vi "test_CCDSetAndGetTriggerIn.vi"(7 "Test should pass":bool=TRUE, 8 "error in":errorcluster, 9 "tear down connection":bool=TRUE, 10 "set-up a connection":bool=TRUE, 11 "device selection":enum16{"monochromator", "CCD", "SCD"}(ring)=enum."CCD") -> (0 "error out":errorcluster)   [LabVIEW 2023]
uses:
  <vilib>/addons/_JKI Toolkits/Caraya/classes/Test/Test.lvclass
  <vilib>/addons/_JKI Toolkits/Caraya/classes/Assert/Assert.lvclass
  <vilib>/addons/_JKI Toolkits/Caraya/classes/Assert/Assert Not Error.vi
  <vilib>/addons/_JKI Toolkits/Caraya/classes/Assert/Assert Equal Value and Type_Variant.vi
  Classes/CCD/CCD.lvclass
  Classes/CCD/TriggerInAddressRing.ctl
  Classes/CCD/TriggerInEventRing.ctl
  Classes/CCD/TriggerInSignalTypeRing.ctl
panel:
  # "Connector Pane"
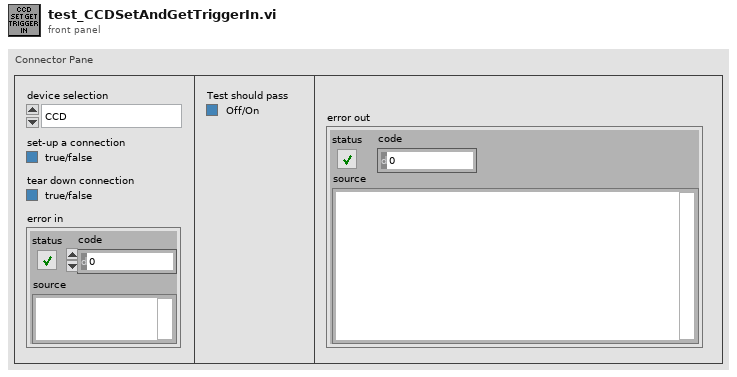
[diagram p1: front panel]
types:
  T1 = typedef "CCD.lvclass/TriggerInSignalTypeRing.ctl" = i32
  T2 = typedef "CCD.lvclass/TriggerInEventRing.ctl" = i32
  T3 = typedef "CCD.lvclass/TriggerInAddressRing.ctl" = i32
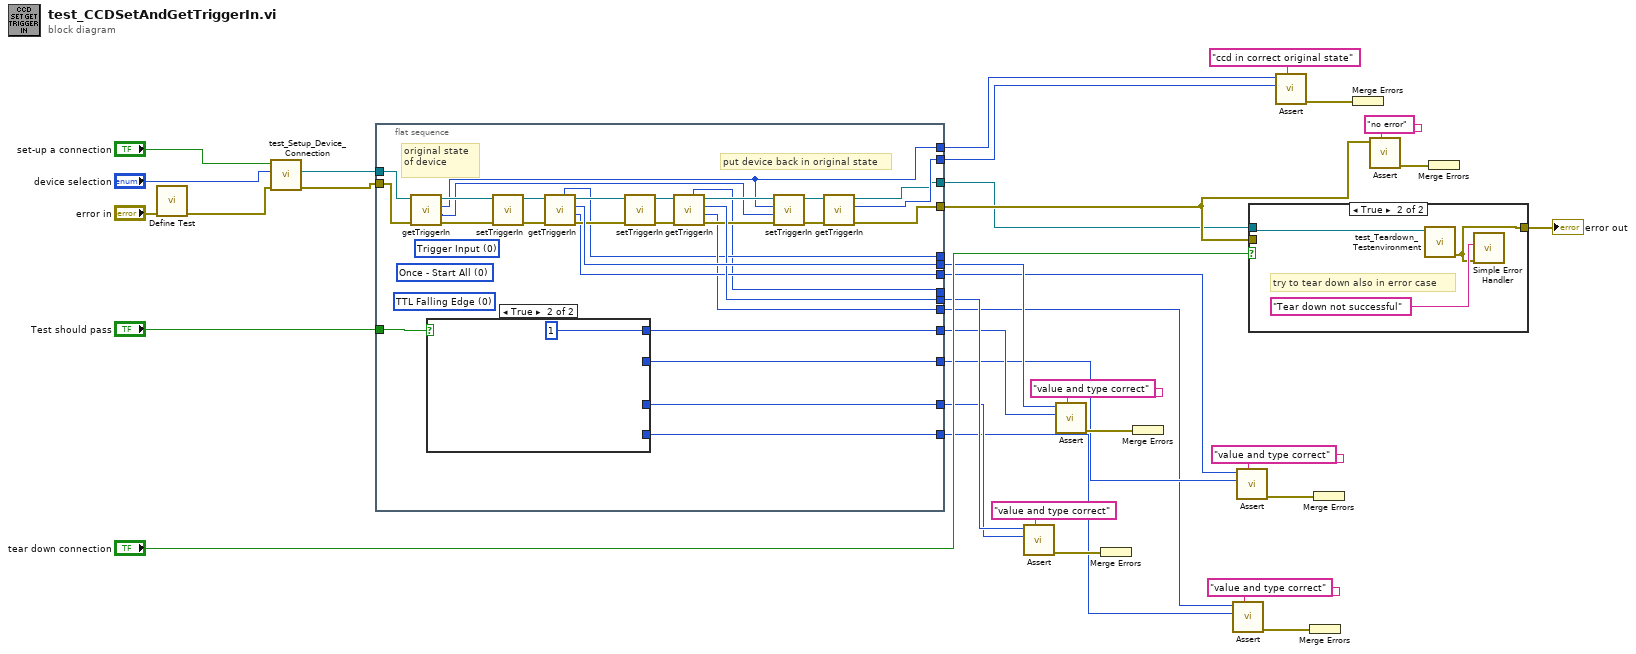
[diagram p0: block diagram]
diagram:
  n1 = call <vilib>:"Define Test.vi"("error in (no error)"="error in") -> ("error out"=w4:errorcluster)  [unwired: 9 in, 1 out]
  n2 = call "test_Setup_Device_Connection.vi"("error in (no error)"=w4, "device selection"="device selection", "set-up a connection"="set-up a connection") -> ("error out"=w5:errorcluster, "CCD out"=w3:refnum<class "CCD.lvclass">)  [unwired: 5 in, 2 out]
  n3 = flat-sequence {
    tunnel: w5 -> [w59]
    tunnel: w3 -> [w60]
    tunnel: [w41] -> w24
    tunnel: "Test should pass" -> [w63]
    tunnel: [w42] -> w23
    tunnel: [w49] -> w22
    tunnel: [w62] -> w21
    tunnel: [w54] -> w20
    tunnel: [w61] -> w19
    tunnel: [w44] -> w16
    tunnel: [w43] -> w15
    tunnel: [w39] -> w11
    tunnel: [w38] -> w10
    tunnel: [w37] -> w7
    tunnel: [w36] -> w6
    tunnel: [w35] -> _
    tunnel: [w34] -> _
    frame #0 {
      (unwired) T1 0 items=["Input Trigger Disabled"=-1, "TTL Falling Edge"=0, "TTL Rising Edge"=1] ("signalType")
      (unwired) T2 0 items=["Input Trigger Disabled"=-1, "Once - Start All"=0, "Each - For Each Acq"=1] ("event")
      (unwired) T3 0 items=["Input Trigger Disabled"=-1, "Trigger Input"=0] ("address")
      # "put device back in original state"
      # "original state of device"
      n4 = call "getTriggerIn.vi"("error in (no error)"=w59, "CCD in"=w60) -> ("error out"=w57:errorcluster, "signalType"=w40:T1, "event"=w44:T2, "CCD out"=w58:refnum<class "CCD.lvclass">)  [unwired: 5 in, 1 out]
      n5 = case shown="True" w63 {
        tunnel: [w64 w69] -> w62
        tunnel: [w66 1 ("exposure time [ms]")] -> w61
        tunnel: [w65 w68] -> w39
        tunnel: [_ w67] -> w36
        frame False {
        }
        frame True {
        }
      }
      n6 = call "setTriggerIn.vi"("error in (no error)"=w57, "CCD in"=w58) -> ("error out"=w56:errorcluster, "CCD out"=w55:refnum<class "CCD.lvclass">)  [unwired: 6 in, 2 out]
      n7 = call "getTriggerIn.vi"("error in (no error)"=w56, "CCD in"=w55) -> ("error out"=w50:errorcluster, "signalType"=w38:T1, "event"=w54:T2, "CCD out"=w51:refnum<class "CCD.lvclass">, "address"=w35:T3)  [unwired: 5 in]
      n8 = call "setTriggerIn.vi"("error in (no error)"=w50, "CCD in"=w51) -> ("error out"=w53:errorcluster, "CCD out"=w52:refnum<class "CCD.lvclass">)  [unwired: 6 in, 2 out]
      n9 = call "getTriggerIn.vi"("error in (no error)"=w53, "CCD in"=w52) -> ("error out"=w46:errorcluster, "signalType"=w37:T1, "event"=w49:T2, "CCD out"=w47:refnum<class "CCD.lvclass">, "address"=w34:T3)  [unwired: 5 in]
      n10 = call "setTriggerIn.vi"("error in (no error)"=w46, "signalType"=w40, "event"=w44, "CCD in"=w47) -> ("error out"=w48:errorcluster, "CCD out"=w45:refnum<class "CCD.lvclass">)  [unwired: 4 in, 2 out]
      n11 = call "getTriggerIn.vi"("error in (no error)"=w48, "CCD in"=w45) -> ("error out"=w41:errorcluster, "event"=w43:T2, "CCD out"=w42:refnum<class "CCD.lvclass">)  [unwired: 5 in, 2 out]
    }
  }
  n12 = call-poly <vilib>:"Assert.vi"("Label"="value and type correct" ("Label (VI Title)"), "Y"=w21, "X"=w22) -> ("error out"=w32:errorcluster)  [unwired: 7 in, 1 out]
  n13 = call-poly <vilib>:"Assert.vi"("Label"="value and type correct" ("Label (VI Title)"), "Y"=w19, "X"=w20) -> ("error out"=w31:errorcluster)  [unwired: 7 in, 1 out]
  n14 = Merge Errors(w32) -> ()  [unwired: 1 out]
  n15 = Merge Errors(w31) -> ()  [unwired: 1 out]
  n16 = call-poly <vilib>:"Assert.vi"("Label"="value and type correct" ("Label (VI Title)"), "Y"=w6, "X"=w7) -> ("error out"=w9:errorcluster)  [unwired: 7 in, 1 out]
  n17 = call-poly <vilib>:"Assert.vi"("Label"="value and type correct" ("Label (VI Title)"), "Y"=w11, "X"=w10) -> ("error out"=w12:errorcluster)  [unwired: 7 in, 1 out]
  n18 = case shown="True" "tear down connection" {
    tunnel: w23 -> [_ w73]
    tunnel: [w71 w72] -> w14
    tunnel: w24 -> [w71 _]
    frame False {
    }
    frame True {
      # "try to tear down also in error case"
      n19 = call "test_Teardown_Testenvironment.vi"("GenericDevice.lvclass"=w73) -> ("error out"=w72:errorcluster)  [unwired: 9 in, 1 out]
      n20 = call <vilib>:"Simple Error Handler.vi"("error source (\" \")"="Tear down not successful" ("error source (\" \")"), "error in (no error)"=w72) -> ()  [unwired: 3 in, 5 out]
    }
  }
  "error out" <- w14
  n21 = call-poly <vilib>:"Assert.vi"("Label"="ccd in correct original state" ("Label (VI Title)"), "Y"=w15, "X"=w16) -> ("error out"=w18:errorcluster)  [unwired: 7 in, 1 out]
  n22 = Merge Errors(w9) -> ()  [unwired: 1 out]
  n23 = Merge Errors(w12) -> ()  [unwired: 1 out]
  n24 = Merge Errors(w18) -> ()  [unwired: 1 out]
  n25 = call-poly <vilib>:"Assert.vi"("Label"="no error" ("Label (VI Title)"), "Not Error?"=w24) -> ("error out"=w26:errorcluster)  [unwired: 8 in, 1 out]
  n26 = Merge Errors(w26) -> ()  [unwired: 1 out]
